vi "AddInterfaceToProject.vi"(8 "error in (no error)":errorcluster, 11 "CreateInterface in":refnum<class "CreateInterface.lvclass">) -> (0 "error out":errorcluster, 3 "CreateInterface out":refnum<class "CreateInterface.lvclass">)   [LabVIEW 2020, in "Mermaid.lvlib" / "CreateInterface.lvclass"]
uses:
  CreateInterface.lvclass
  CreateInterface.lvclass/CreateInterface.ctl
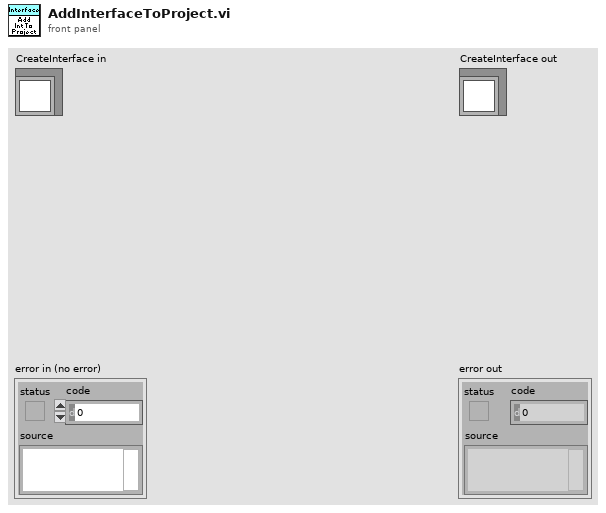
[diagram p1: front panel]
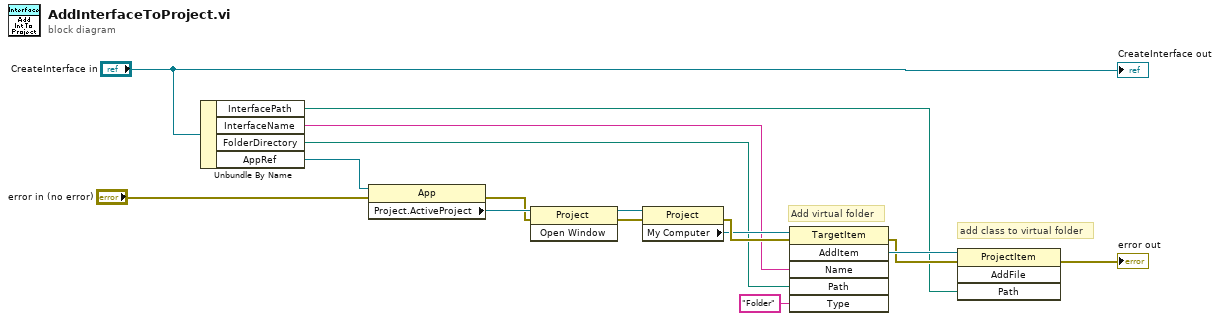
[diagram p0: block diagram]
diagram:
  # "add class to virtual folder"
  # "Add virtual folder"
  n1 = Unbundle By Name("CreateInterface in") -> ("InterfacePath"=w3:path, "InterfaceName"=w1:string, "FolderDirectory"=w2:path, "AppRef"=w4:refnum<vi>)
  n2 = property class="App"(reference=w4, error in="error in (no error)") -> (error out=w10:errorcluster, "Project.ActiveProject"=w11:refnum<vi>)  [unwired: 1 out]
  n3 = invoke class="Project" method="Open Window"(reference=w11, error in=w10) -> (reference out=w14:refnum<vi>, error out=w13:errorcluster)  [unwired: 1 in, 1 out]
  n4 = property class="Project"(reference=w14, error in=w13) -> (error out=w16:errorcluster, "My Computer"=w12:refnum<vi>)  [unwired: 1 out]
  n5 = invoke class="TargetItem" method="AddItem"(reference=w12, error in=w16, "Name"=w1, "Path"=w2, "Type"="Folder") -> (error out=w8:errorcluster, "AddItem"=w9:refnum<vi>)  [unwired: 1 in, 4 out]
  n6 = invoke class="ProjectItem" method="AddFile"(reference=w9, error in=w8, "Path"=w3) -> (error out=→"error out":errorcluster)  [unwired: 1 in, 3 out]
  "CreateInterface out" <- "CreateInterface in"
